vi "Check.vi"(11 "Timer in":refnum<class "Timer.lvclass">) -> (1 "Name":string, 2 "Elapsed":bool, 3 "Timer out":refnum<class "Timer.lvclass">, 4 "Metadata":string)   [LabVIEW 2015, in "Timer.lvclass"]
doc: "Checks to see if a Task has become due (i.e. the time since the Event last occured is greater than the Task Period).\n\nIf the Task is due, then the elapsed time is reset and the User Event associated with this Task is fired off."
uses:
  Timer.lvclass
  Timer.lvclass/Timer.ctl
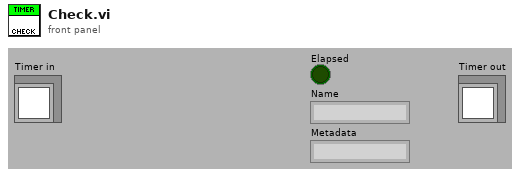
[diagram p1: front panel]
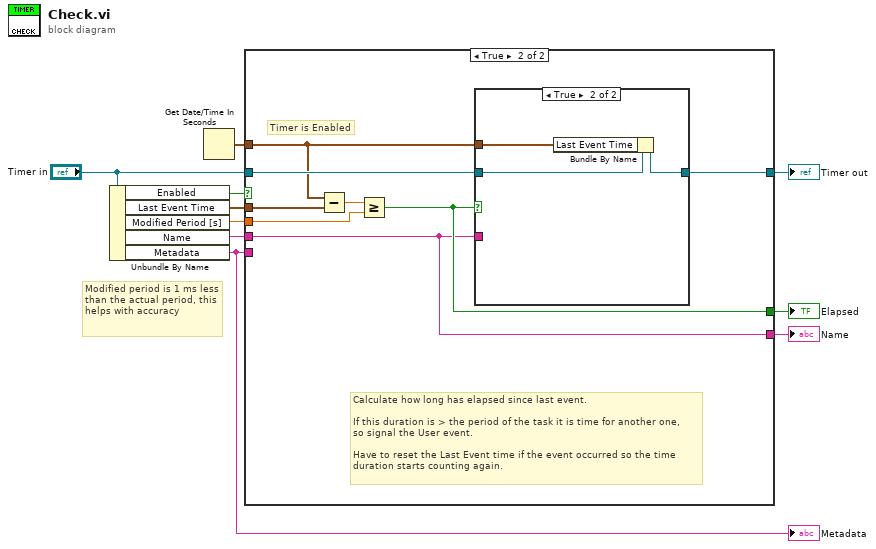
[diagram p0: block diagram]
diagram:
  # "Modified period is 1 ms less than the actual period, this helps with accuracy"
  n1 = Unbundle By Name("Timer in") -> ("Enabled"=w3:bool, "Last Event Time"=w2:timestamp, "Modified Period [s]"=w8:dbl, "Name"=w7:string, "Metadata"=w1:string)
  "Metadata" <- w1
  n2 = Get Date/Time In Seconds() -> (seconds since 1Jan1904=w6:timestamp)
  n3 = case shown="True" w3 {
    tunnel: w8 -> [_ w13]
    tunnel: "Timer in" -> [w11 w19]
    tunnel: [w11 w18] -> w9
    tunnel: w7 -> [_ w14]
    tunnel: w6 -> [_ w16]
    tunnel: [_ w15] -> w5
    tunnel: [_ w14] -> w4
    tunnel: w2 -> [_ w12]
    tunnel: w1 -> [_ _]
    frame False {
      # "Timer is not active. No action necessary."
    }
    frame True {
      # "Timer is Enabled"
      # "Calculate how long has elapsed since last event.\n\nIf this duration is > the period of the task it is time for another one,\nso signal the User event.\n\nHave to reset the Last Event time if the event occurred so the time\nduration starts counting again."
      n4 = Subtract(x=w16, y=w12) -> (x-y=w17:dbl)
      n5 = Greater Or Equal?(x=w17, y=w13) -> (x >= y?=w15:bool)
      n6 = case shown="True" w15 {
        tunnel: w19 -> [w20 w23]
        tunnel: [w20 w22] -> w18
        tunnel: w14 -> [_ _]
        tunnel: w16 -> [_ w21]
        frame False {
        }
        frame True {
          n7 = Bundle By Name(cluster=w23, "Last Event Time"=w21) -> (w22:refnum<class "Timer.lvclass">)
        }
      }
    }
  }
  "Timer out" <- w9
  "Elapsed" <- w5
  "Name" <- w4
